vi "publish -- magnet -- DC -- V2.vi"(7 "publisher action":T2, 10 "Array":T1[](array[typedef])) -> (2 "Array OUT":T1[](array[typedef]))   [LabVIEW 2019]
uses:
  publisher action.ctl
  icicle.ctl
panel:
  in  "Field IN (T)":dbl=1000.0 format="%#_10f"
  out "Field out (T)":dbl=1000.0 format="%#_10f"
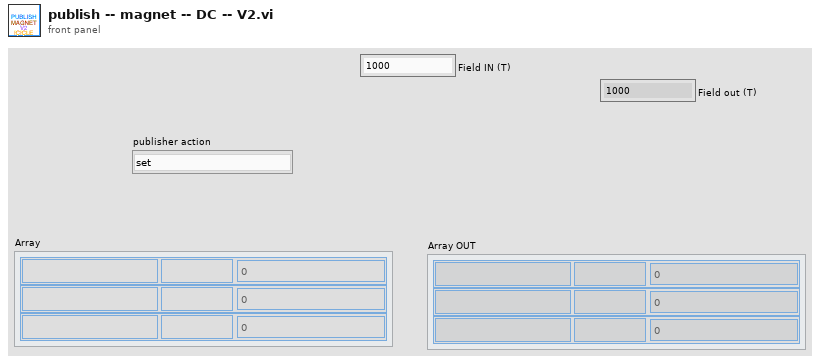
[diagram p1: front panel]
types:
  T1 = typedef "icicle.ctl" = cluster{"name":string, "units":string, "data":dbl}
  T2 = typedef "publisher action.ctl" = enum16{"set", "get", "init", "check"}
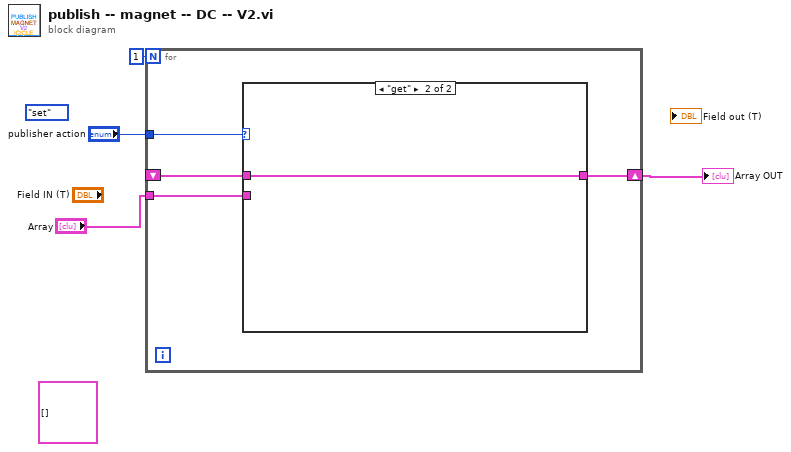
[diagram p0: block diagram]
diagram:
  (unwired) T1[] [] ("Array")
  (unwired) publisher_action."set" ("publisher action")
  n1 = for {
    N: 1 -> [_]
    tunnel: "publisher action" -> [w8]
    tunnel: "Array" -> [w6]
    shift-right: [w7] -> w1
    shift-left: _ -> [w5]
    n2 = case shown="\"get\"" w8 {
      tunnel: [w9 w10] -> w7
      tunnel: w6 -> [w9 _]
      tunnel: w5 -> [_ w10]
      frame "set", Default {
      }
      frame "get" {
      }
    }
  }
  "Array OUT" <- w1
